vi "Low's Mutation.vi"(11 "Schedule":u16[](array[numeric])) -> (3 "Mutated Solution":u16[](array[numeric]))   [LabVIEW 2013, in "GA.lvclass"]
uses:
  GA.lvclass
panel:
  out "Index 2":i32
  out "Index 1":i32
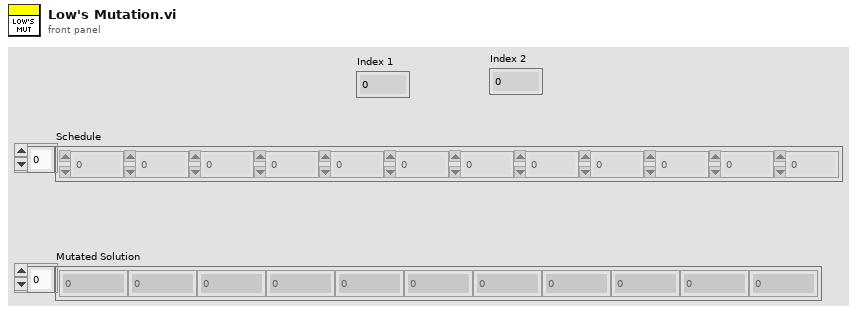
[diagram p1: front panel]
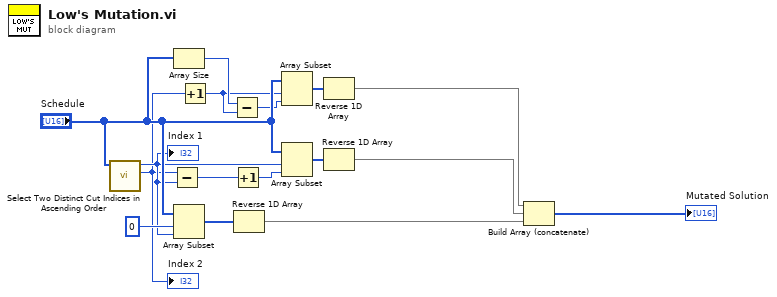
[diagram p0: block diagram]
diagram:
  n1 = call "Select Two Distinct Cut Indices in Ascending Order.vi"("Schedule"="Schedule") -> ("Index 2"=w8:i32, "Index 1"=w13:i32)  [unwired: 9 in]
  "Index 1" <- w13
  "Index 2" <- w8
  n2 = Subtract(x=w8, y=w13) -> (x-y=w12:i32)
  n3 = Array Size(array="Schedule") -> (size(s)=w9:i32)
  n4 = Array Subset(array="Schedule", index=0, length=w13) -> (w15:u16[])
  n5 = Increment(x=w8) -> (x+1=w7:i32)
  n6 = Subtract(x=w9, y=w7) -> (x-y=w6:i32)
  n7 = Increment(x=w12) -> (x+1=w11:i32)
  n8 = Reverse 1D Array(array=w15) -> (reversed array=w1:u16[])
  n9 = Array Subset(array="Schedule", index=w7, length=w6) -> (w5:u16[])
  n10 = Array Subset(array="Schedule", index=w13, length=w11) -> (w10:u16[])
  n11 = Reverse 1D Array(array=w5) -> (reversed array=w2:u16[])
  n12 = Reverse 1D Array(array=w10) -> (reversed array=w4:u16[])
  n13 = Build Array (concatenate)(w2, w4, w1) -> (→"Mutated Solution":u16[])
